vi "gyroNumControl.vi"() -> ()   [LabVIEW 2017]
panel:
  in  "gyro":dbl
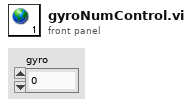
[diagram p1: front panel]
diagram:
